vi "Actor Core.vi"(8 "error in":errorcluster, 11 "Limites Contador in":refnum<class "Limites Contador.lvclass">) -> (0 "error out":errorcluster, 3 "Actor out":refnum<class "Actor.lvclass">)   [LabVIEW 2020, in "Limites Contador.lvlib" / "Limites Contador.lvclass"]
doc: "(<B>Filename</B>: Actor Framework.lvlib:Actor.lvclass:Actor Core.vi)\n\nReceives messages to the actor, reacts to them, and initiates any error handling that may shut the actor down.\n\nDescendant classes may override this VI to append parallel tasks for the actor to complete while it handles messages. Overrides use the Call Parent Class Method node."
uses:
  Limites Contador.lvclass
  C:/Program Files (x86)/National Instruments/LabVIEW 2020/vi.lib/ActorFramework/Actor/Actor.lvclass
  <vilib>/ActorFramework/Actor/Actor.lvclass
  <vilib>/ActorFramework/Actor/Actor.lvclass/Actor.ctl
  Limites Contador.lvclass/Limites Contador.ctl
  GUI DigitalCount Messages/Final Count Msg/Final Count Msg.lvclass/Final Count Msg.ctl
  <vilib>/ActorFramework/Message Enqueuer/Message Enqueuer.lvclass/Message Enqueuer.ctl
  <vilib>/ActorFramework/Message Enqueuer/Enqueue.vi
  GUI DigitalCount Messages/Final Count Msg/Final Count Msg.lvclass
  C:/Program Files (x86)/National Instruments/LabVIEW 2020/vi.lib/ActorFramework/Message/Message.lvclass
  <vilib>/ActorFramework/Message Priority Queue/Priority Enqueue.vi
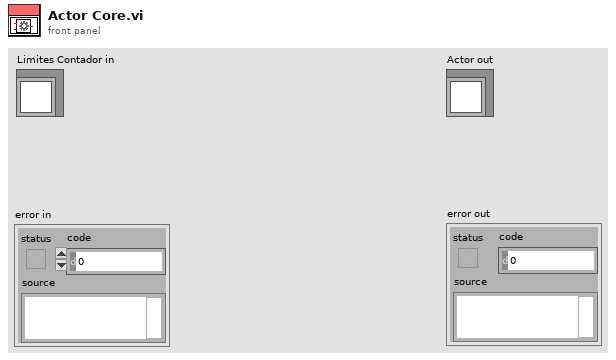
[diagram p1: front panel]
types:
  T1 = cluster{"Limit Superior":dbl, "Limit Inferior":dbl, "Numero Actual":dbl}
  T2 = cluster{"Start/stop Event":refnum<user-event>, "Exit Event":refnum<user-event>, "Limites Event":refnum<user-event>}
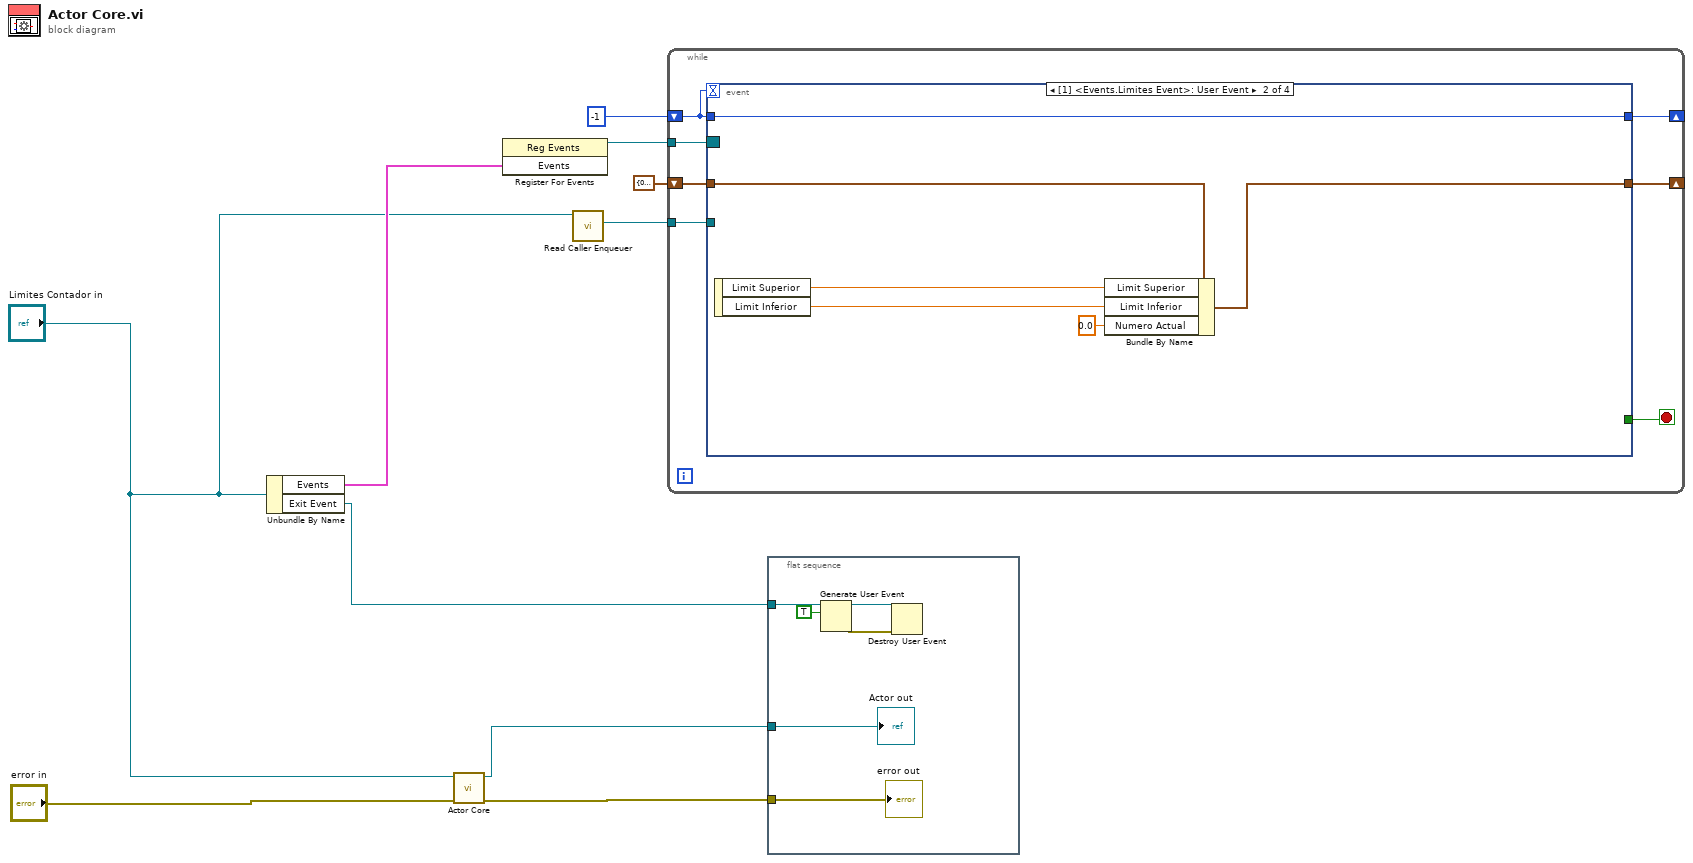
[diagram p0: block diagram]
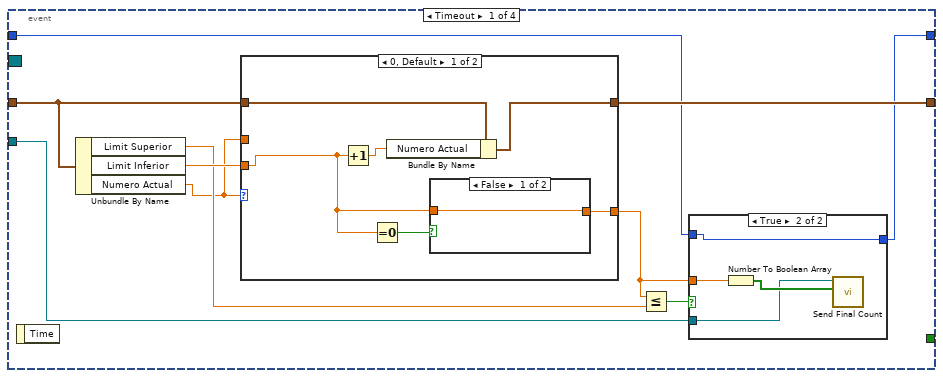
[diagram p2: hidden frame]
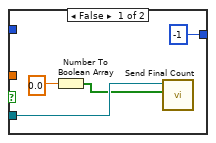
[diagram p3: hidden frame]
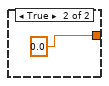
[diagram p4: hidden frame]
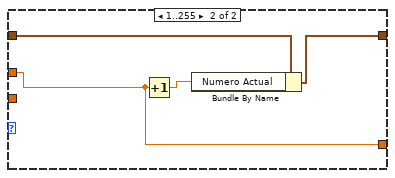
[diagram p5: hidden frame]
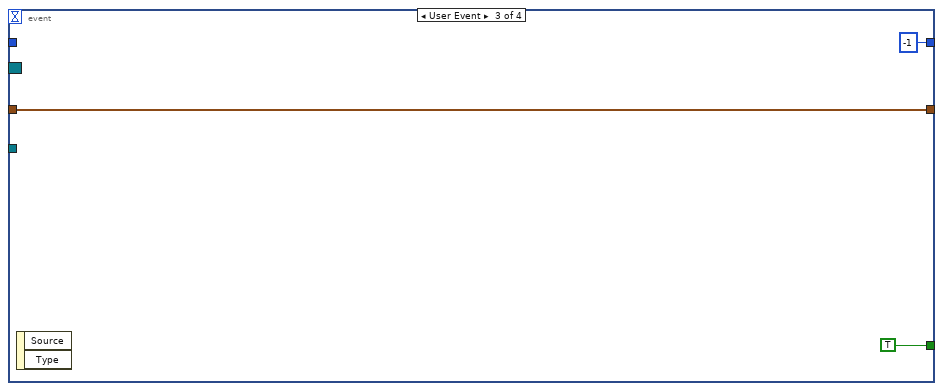
[diagram p6: hidden frame]
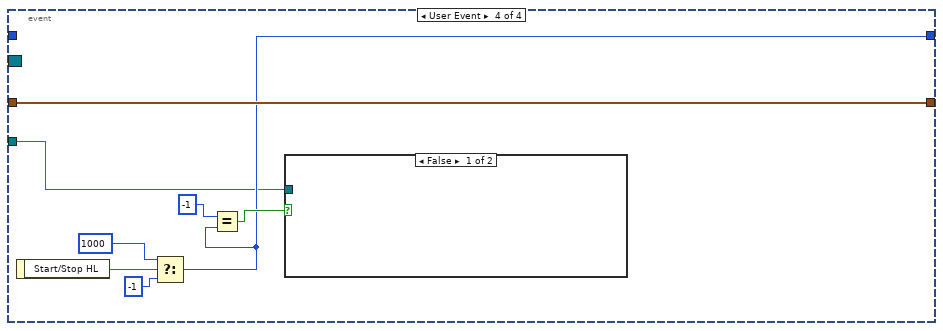
[diagram p7: hidden frame]
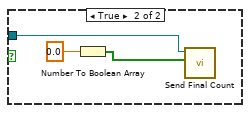
[diagram p8: hidden frame]
diagram:
  n1 = Unbundle By Name("Limites Contador in") -> ("Events"=w6:T2, "Exit Event"=w7:refnum<user-event>)
  n2 = call-parent "Actor Core.vi"("error in"="error in", "Actor in"="Limites Contador in") -> ("error out"=w10:errorcluster, "Actor out"=w9:refnum<class "Actor.lvclass">)  [unwired: 8 in]
  n3 = register-events(w6) -> (reference out=w3:refnum<event-registration>)  [unwired: 2 in, 1 out]
  n4 = call <vilib>:"Read Caller Enqueuer.vi"("Actor"="Limites Contador in") -> ("Caller Enqueuer"=w1:refnum<class "Message Enqueuer.lvclass">)  [unwired: 10 in]
  n5 = while {
    shift-right: [w16] -> _
    shift-left: -1 -> [w17]
    tunnel: w3 -> [w15]
    shift-right: [w13] -> _
    shift-left: T1 {"Limit Superior"=0.0, "Limit Inferior"=0.0, "Numero Actual"=0.0} ("Limites") -> [w14]
    tunnel: w1 -> [w12]
    stop <- w11 stop-if-true
    n6 = event shown="[1] <Events.Limites Event>: User Event" {
      selector: w15 -> [_ _ _ _]
      dyn-events: _ -> [_ _ _ _]
      timeout: w17 -> [_ _ _ _]
      tunnel: w17 -> [w20 w53 _ _]
      tunnel: [w22 w53 -1 w58] -> w16
      tunnel: [w26 w51 w56 w64] -> w13
      tunnel: w14 -> [w27 w52 w56 w64]
      tunnel: w12 -> [w21 _ _ w57]
      tunnel: [_ _ TRUE _] -> w11
      event Timeout {
        n7 = event-data() -> ()  [unwired: 1 in, 1 out]
        n8 = Unbundle By Name(w27) -> ("Limit Superior"=w24:dbl, "Limit Inferior"=w25:dbl, "Numero Actual"=w18:dbl)
        n9 = case shown="0, Default" w18 {
          tunnel: w27 -> [w41 w47]
          tunnel: [w40 w46] -> w26
          tunnel: w25 -> [w37 _]
          tunnel: [w36 w44] -> w19
          tunnel: w18 -> [_ w44]
          frame 0, Default {
            n10 = Increment(x=w37) -> (x+1=w39:dbl)
            n11 = Equal To 0?(x=w37) -> (x = 0?=w38:bool)
            n12 = Bundle By Name(cluster=w41, "Numero Actual"=w39) -> (w40:T1)
            n13 = case shown="False" w38 {
              tunnel: w37 -> [w42 _]
              tunnel: [w42 0.0] -> w36
              frame False {
              }
              frame True {
              }
            }
          }
          frame 1..255 {
            n14 = Increment(x=w44) -> (x+1=w45:dbl)
            n15 = Bundle By Name(cluster=w47, "Numero Actual"=w45) -> (w46:T1)
          }
        }
        n16 = Less Or Equal?(x=w19, y=w24) -> (x <= y?=w23:bool)
        n17 = case shown="True" w23 {
          tunnel: [-1 w34] -> w22
          tunnel: w21 -> [w30 w33]
          tunnel: w20 -> [_ w34]
          tunnel: w19 -> [_ w32]
          frame False {
            n18 = Number To Boolean Array(number=0.0) -> (Boolean array=w28:bool[])
            n19 = call "Send Final Count.vi"("event data"=w28, "Message Enqueuer"=w30) -> ()  [unwired: 8 in, 2 out]
          }
          frame True {
            n20 = Number To Boolean Array(number=w32) -> (Boolean array=w35:bool[])
            n21 = call "Send Final Count.vi"("event data"=w35, "Message Enqueuer"=w33) -> ()  [unwired: 8 in, 2 out]
          }
        }
      }
      event User Event {
        n22 = event-data() -> ("Limit Superior"=w50:dbl, "Limit Inferior"=w49:dbl)  [unwired: 1 in]
        n23 = Bundle By Name(cluster=w52, "Limit Superior"=w50, "Limit Inferior"=w49, "Numero Actual"=0.0) -> (w51:T1)
      }
      event User Event {
        n24 = event-data() -> ()  [unwired: 1 in, 2 out]
      }
      event User Event {
        n25 = event-data() -> ("Start/Stop HL"=w63:bool)  [unwired: 1 in]
        n26 = Select(t=1000, s=w63, f=-1) -> (s? t:f=w58:i32)
        n27 = Equal?(x=-1, y=w58) -> (x = y?=w59:bool)
        n28 = case shown="False" w59 {
          tunnel: w57 -> [_ w66]
          frame False {
          }
          frame True {
            n29 = Number To Boolean Array(number=0.0) -> (Boolean array=w67:bool[])
            n30 = call "Send Final Count.vi"("event data"=w67, "Message Enqueuer"=w66) -> ()  [unwired: 8 in, 2 out]
          }
        }
      }
    }
  }
  n31 = flat-sequence {
    tunnel: w10 -> [w73]
    tunnel: w9 -> [w72]
    tunnel: w7 -> [w69]
    frame #0 {
      n32 = Generate User Event(user event=w69, event data cluster=TRUE ("event data")) -> (user event out=w71:refnum<user-event>, error out=w70:errorcluster)  [unwired: 2 in]
      n33 = Destroy User Event(user event=w71, error in=w70) -> ()  [unwired: 1 out]
      "error out" <- w73
      "Actor out" <- w72
    }
  }
